vi "Save to RAW TDMS.vi"(8 "error in (no error)":errorcluster, 11 "Scan Data Process":T1) -> (0 "error out":errorcluster, 3 "Scan Data Process out":T1)   [LabVIEW 2015, in "Exposure Process.lvlib"]
uses:
  Exposure Process.lvlib
  Control_Scan Data Process.ctl
  <vilib>/addons/PointValueMap/controls/PointMap.ctl
  Control_EXP Information.ctl
  Control_File Save Setup.ctl
  Control_Enable and Path.ctl
  Control_ICM Export Setting.ctl
  FileHandler/controls/Record.ctl
  FileHandler/FileHandler.lvlib
  <vilib>/addons/PointValueMap/PointValueMap.lvlib
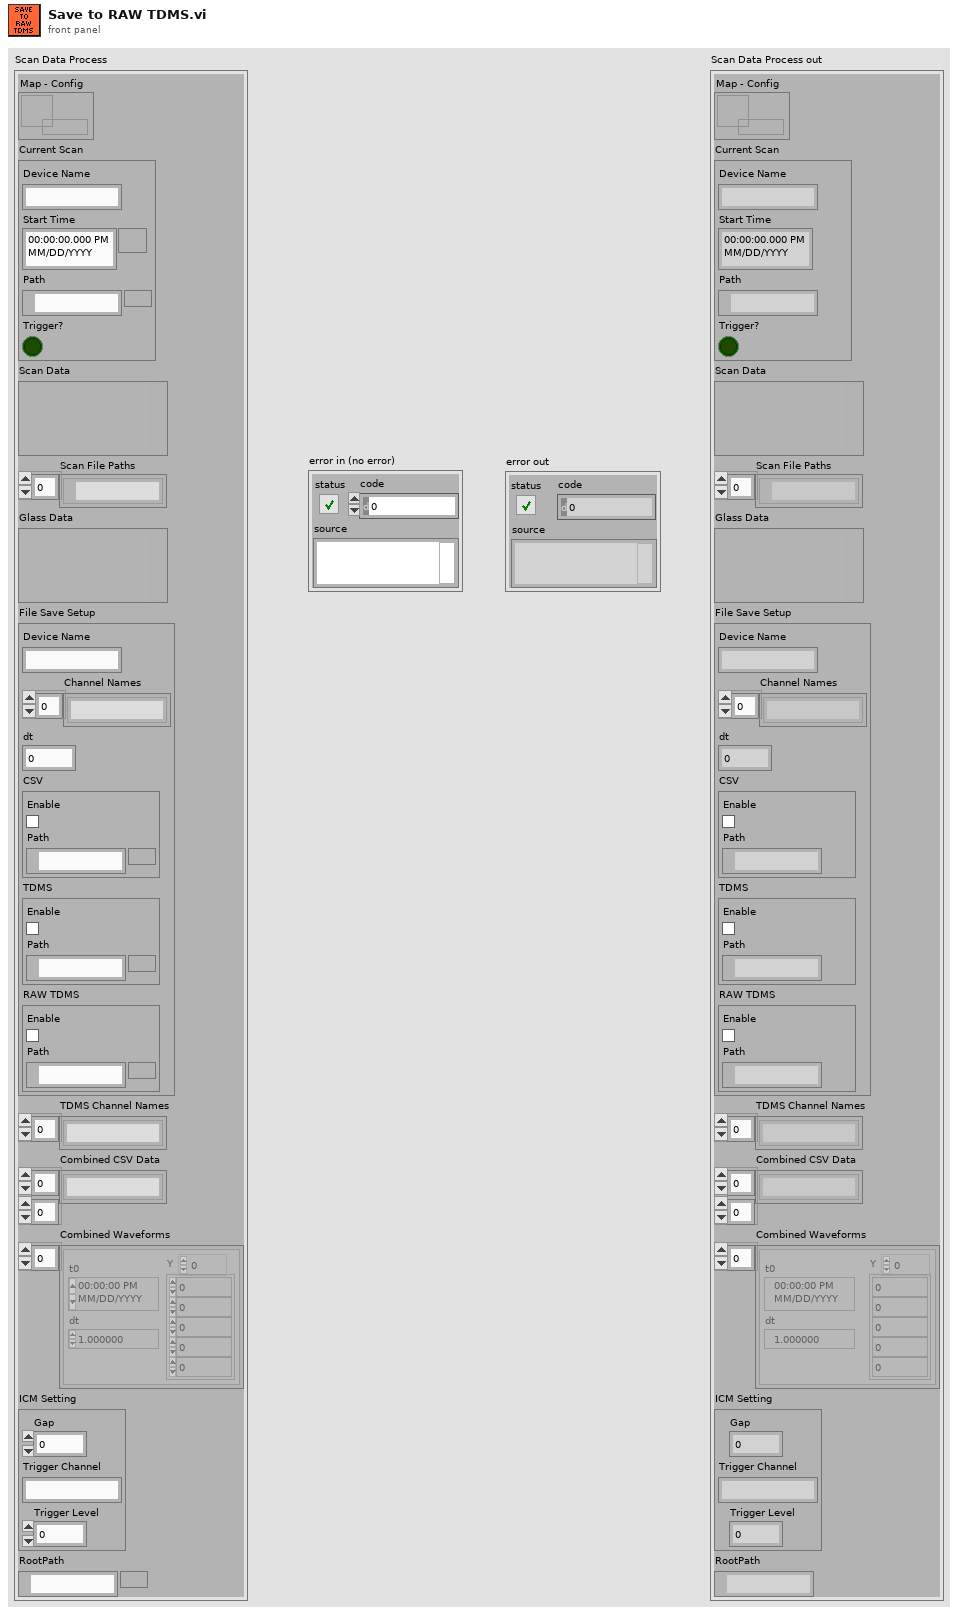
[diagram p1: front panel]
types:
  T1 = typedef "Exposure Process.lvlib/Control_Scan Data Process.ctl" = cluster{"Map - Config":T2, "Current Scan":T3, "Scan Data":variant, "Scan File Paths":path[], "Glass Data":variant, "File Save Setup":T4, "TDMS Channel Names":string[], "Combined CSV Data":string[][], "Combined Waveforms":waveform(dbl)[], "ICM Setting":T6, "RootPath":path}
  T2 = typedef "PointValueMap.lvlib/PointMap.ctl" = refnum<data-value>
  T3 = typedef "Exposure Process.lvlib/Control_EXP Information.ctl" = cluster{"Device Name":string, "Start Time":timestamp, "Path":path, "Trigger?":bool}
  T4 = typedef "Exposure Process.lvlib/Control_File Save Setup.ctl" = cluster{"Device Name":string, "Channel Names":string[], "dt":dbl, "CSV":T5, "TDMS":T5, "RAW TDMS":T5}
  T5 = typedef "Exposure Process.lvlib/Control_Enable and Path.ctl" = cluster{"Enable":bool, "Path":path}
  T6 = typedef "Exposure Process.lvlib/Control_ICM Export Setting.ctl" = cluster{"Gap":dbl, "Trigger Channel":string, "Trigger Level":dbl}
  T7 = typedef "FileHandler.lvlib/Record.ctl" = cluster{"Time":timestamp, "Path":path}
  T8 = enum16{"open", "open or create", "create or replace", "create", "open (read-only)"}
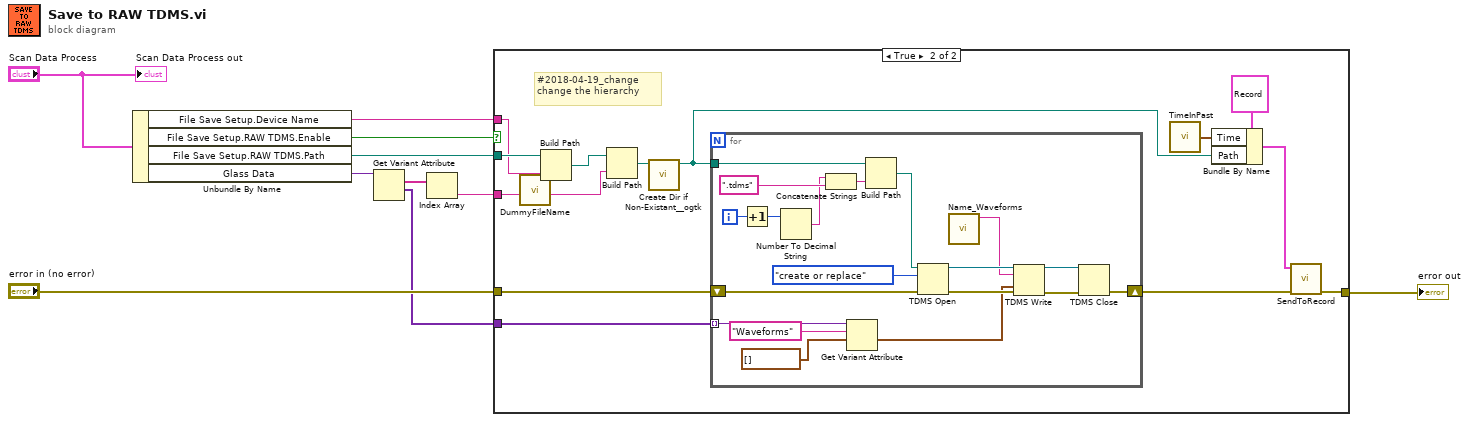
[diagram p0: block diagram]
diagram:
  n1 = Unbundle By Name("Scan Data Process") -> ("File Save Setup.Device Name"=w1:string, "File Save Setup.RAW TDMS.Enable"=w9:bool, "File Save Setup.RAW TDMS.Path"=w8:path, "Glass Data"=w7:variant)
  n2 = Get Variant Attribute(Variant=w7) -> (names=w6:string[], values=w3:variant[])  [unwired: 3 in, 2 out]
  n3 = Index Array(array=w6) -> (element=w5:string)  [unwired: 1 in]
  n4 = case shown="True" w9 {
    tunnel: "error in (no error)" -> [w11 w25]
    tunnel: [w11 w14] -> w10
    tunnel: w8 -> [_ w21]
    tunnel: w3 -> [_ w24]
    tunnel: w5 -> [_ w22]
    tunnel: w1 -> [_ w19]
    frame False {
    }
    frame True {
      # "#2018-04-19_change\nchange the hierarchy"
      n5 = call "DummyFileName.vi"("Time String in"=w22) -> ("Time String out"=w12:string)  [unwired: 9 in, 1 out]
      n6 = Build Path(base path=w21, name or relative path=w19) -> (appended path=w20:path)
      n7 = Build Path(base path=w20, name or relative path=w12) -> (appended path=w23:path)
      n8 = call <userlib>:"Create Dir if Non-Existant__ogtk.vi"("Directory Path"=w23) -> ("dup Directory Path"=w13:path)  [unwired: 8 in, 2 out]
      n9 = for {
        shift-right: [w38] -> w15
        shift-left: w25 -> [w43]
        tunnel: w13 -> [w36]
        tunnel: w24 -> [w32] mode=indexing
        i -> [w28]
        n10 = Increment(x=w28) -> (x+1=w27:i32)
        n11 = Number To Decimal String(number=w27) -> (decimal integer string=w26:string)  [unwired: 1 in]
        n12 = Concatenate Strings(w26, ".tdms" ("string")) -> (w34:string)
        n13 = Get Variant Attribute(Variant=w32, name="Waveforms", default value (empty Variant)=waveform(dbl)[] []) -> (value=w29:waveform(dbl)[])  [unwired: 1 in, 3 out]
        n14 = Build Path(base path=w36, name or relative path=w34) -> (appended path=w33:path)
        n15 = TDMS Open(8:w43, 10:T8."create or replace" ("operation (0:open)"), 11:w33) -> (0:w41:errorcluster, 3:w42:refnum<k34>)  [unwired: 4 in]
        n16 = call "Name_Waveforms.vi"() -> ("Name"=w37:string)  [unwired: 11 in]
        n17 = TDMS Write(0:w42, 5:w37, 9:w29, 11:w41) -> (4:w40:refnum<k34>, 15:w39:errorcluster)  [unwired: 2 in, 2 out]
        n18 = TDMS Close(8:w39, 11:w40) -> (0:w38:errorcluster)  [unwired: 1 out]
      }
      n19 = call "TimeInPast.vi"() -> ("Time Stamp"=w18:timestamp)
      n20 = Bundle By Name(cluster=T7 {"Time"=timestamp(0 s since 1904-01-01), "Path"=path ""} ("Record"), "Time"=w18, "Path"=w13) -> (w17:T7)
      n21 = call "SendToRecord.vi"("error in (no error)"=w15, "Record"=w17) -> ("error out"=w14:errorcluster)  [unwired: 9 in]
    }
  }
  "error out" <- w10
  "Scan Data Process out" <- "Scan Data Process"
